vi "p2.vi"() -> ()   [LabVIEW 2021, in "d3.lvlib"]
uses:
  d3.lvlib
  <vilib>/regexp/Match Regular Expression.xnode
  AOC/AOC.lvlib
panel:
  in  "Example":string="vJrwpWtwJgWrhcsFMMfFFhFp\njqHRNqRjqzjGDLGLrsFMfFZSrLrFZsSL\nPmmdzqPrVvPwwTWBwg\nwMqvLMZHhHMvwLHjbvcjnnSBnvTQFn\nttgJtRGJQctTZtZT\nCrZsJsPPZsGzwwsLwLmpwMDw"
  in  "Example":bool
  out "Answer":i64=2604
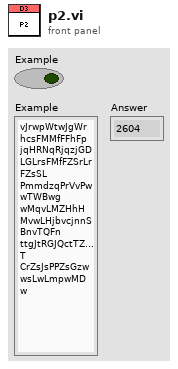
[diagram p1: front panel]
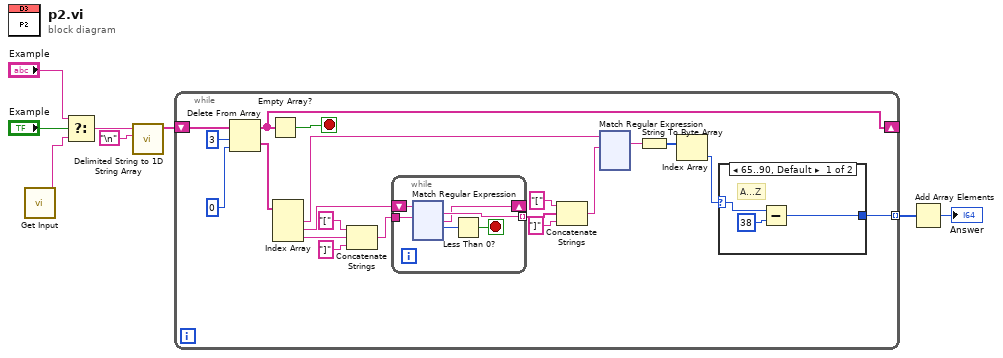
[diagram p0: block diagram]
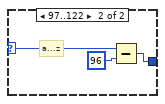
[diagram p2: hidden frame]
diagram:
  n1 = call "Get Input.vi"() -> ("Input"=w6:string)  [unwired: 11 in]
  n2 = Select(t="Example", s="Example", f=w6) -> (s? t:f=w5:string)
  n3 = call <vilib>:"Delimited String to 1D String Array.vi"("delimiter"="\n", "delimited string"=w5) -> ("string array"=w3:string[])  [unwired: 9 in]
  n4 = while {
    tunnel: [w26] -> w7 mode=indexing
    shift-right: [w16] -> _
    shift-left: w3 -> [w25]
    stop <- w15 stop-if-true
    n5 = Delete From Array(array=w25, length=3, index=0) -> (deleted portion=w22:string[], array with subset deleted=w16:string[])
    n6 = Empty Array?(array=w16) -> (empty?=w15:bool)
    n7 = Index Array(array=w22) -> (element #1=w18:string, element #2=w10:string, element #3=w11:string)  [unwired: 3 in]
    n8 = Concatenate Strings("[" ("string"), w11, "]" ("string")) -> (w12:string)
    n9 = while {
      tunnel: w12 -> [w34]
      tunnel: [w32] -> w9 mode=indexing
      shift-right: [w31] -> _
      shift-left: w10 -> [w33]
      stop <- w29 stop-if-true
      n10 = xnode "Match Regular Expression"("input string"=w33, "regular expression"=w34) -> ("whole match"=w32:string, "after match"=w31:string, "offset past match"=w30:i32)  [unwired: 4 in, 2 out]
      n11 = Less Than 0?(x=w30) -> (x < 0?=w29:bool)
    }
    n12 = Concatenate Strings("[" ("string"), w9, "]" ("string")) -> (w19:string)
    n13 = xnode "Match Regular Expression"("input string"=w18, "regular expression"=w19) -> ("whole match"=w17:string)  [unwired: 4 in, 4 out]
    n14 = String To Byte Array(string=w17) -> (unsigned byte array=w28:u8[])
    n15 = Index Array(array=w28) -> (element=w27:u8)  [unwired: 1 in]
    n16 = case shown="65..90, Default" w27 {
      selector: w27 -> [w271 w274]
      tunnel: [w269 w272] -> w26
      frame 65..90, Default {
        # "A...Z"
        n17 = Subtract(x=w271, y=u64 38) -> (x-y=w269:u64)
      }
      frame 97..122 {
        # "a...z"
        n18 = Subtract(x=w274, y=u8 96) -> (x-y=w272:u8)
      }
    }
  }
  n19 = Add Array Elements(numeric array=w7) -> (sum=→"Answer":u64)
